vi "LNLS FOFB Config to FOFBC.vi"(8 "error in (no error)":errorcluster, 11 "LNLS Control FOFB Configuration Out":T1) -> (0 "error out":errorcluster, 3 "LNLS Control FOFB Configuration Out / PFOFBC Data":T1)   [LabVIEW 2011]
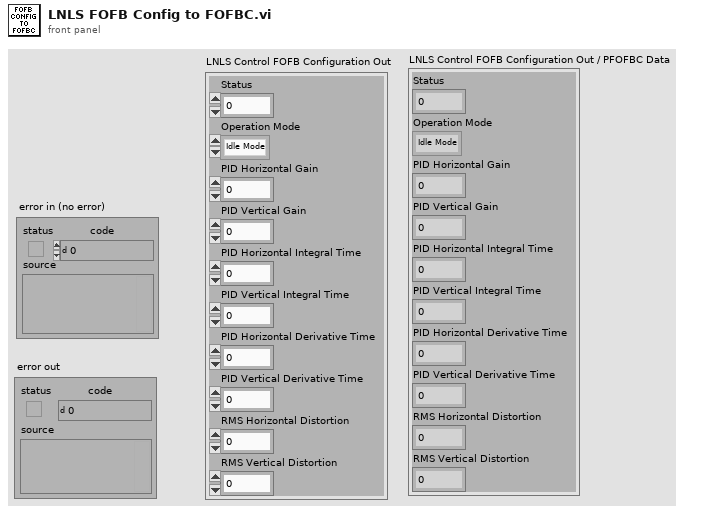
[diagram p1: front panel]
types:
  T1 = cluster{"Status":u16, "Operation Mode":enum8{"Idle Mode", "Error Mode", "Manual Mode", "FOFB Mode", "RMM Mode"}, "PID Horizontal Gain":sgl, "PID Vertical Gain":sgl, "PID Horizontal Integral Time":sgl, "PID Vertical Integral Time":sgl, "PID Horizontal Derivative Time":sgl, "PID Vertical Derivative Time":sgl, "RMS Horizontal Distortion":dbl, "RMS Vertical Distortion":dbl}
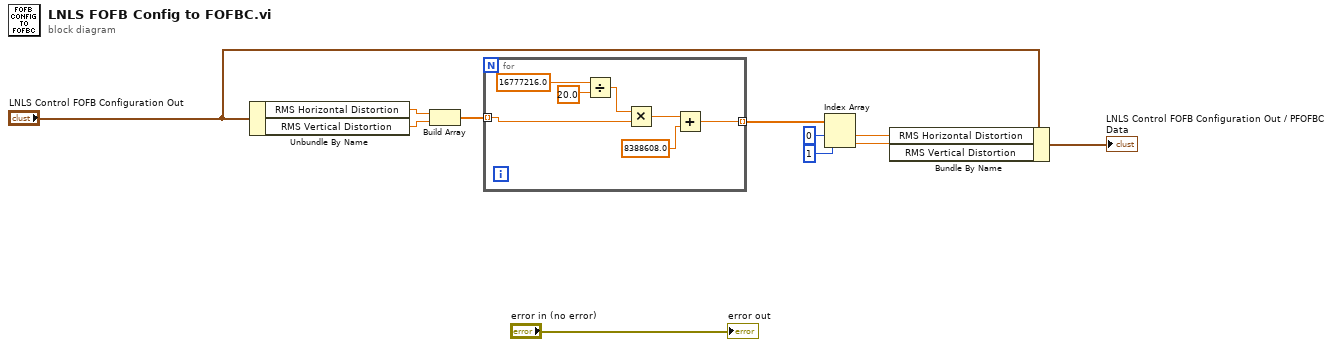
[diagram p0: block diagram]
diagram:
  n1 = Unbundle By Name("LNLS Control FOFB Configuration Out") -> ("RMS Horizontal Distortion"=w6:dbl, "RMS Vertical Distortion"=w7:dbl)
  n2 = Build Array(w6, w7) -> (w8:dbl[])
  n3 = for {
    tunnel: w8 -> [w13] mode=indexing
    tunnel: [w12] -> w9 mode=indexing
    n4 = Divide(x=16777216.0, y=20.0) -> (x/y=w14:dbl)
    n5 = Multiply(x=w14, y=w13) -> (x*y=w18:dbl)
    n6 = Add(x=w18, y=8388608.0) -> (x+y=w12:dbl)
  }
  n7 = Index Array(array=w9, index #1=0 ("index"), index #2=1 ("index")) -> (element #1=w3:dbl, element #2=w2:dbl)
  n8 = Bundle By Name(cluster="LNLS Control FOFB Configuration Out", "RMS Horizontal Distortion"=w3, "RMS Vertical Distortion"=w2) -> (→"LNLS Control FOFB Configuration Out / PFOFBC Data":T1)
  "error out" <- "error in (no error)"
